vi "Get Channels from Stream Names.vi"(8 "error in (no error)":errorcluster, 10 "Stream Names":string[](array[string]), 11 "Sift Stream in":refnum<class "Sift Stream.lvclass">) -> (0 "error out":errorcluster, 2 "Channels":refnum<class "Channel.lvclass">[](array[class]), 3 "Sift Stream out":refnum<class "Sift Stream.lvclass">)   [LabVIEW 2024, in "Sift Stream.lvlib" / "Sift Stream.lvclass"]
uses:
  Sift Stream.lvclass
  <vilib>/FlexLogger/SDK/PluginSDK.lvlibp/PEFClasses/SDK/Channel/Channel.lvclass
  <vilib>/FlexLogger/SDK/PluginSDK.lvlibp/PEFClasses/SDK/Consumer Channel/Consumer Channel.lvclass
  C:/Program Files/National Instruments/LabVIEW 2024/vi.lib/FlexLogger/SDK/PluginSDK.lvlibp/PEFClasses/SDK/Channel/Channel.lvclass
  <vilib>/FlexLogger/SDK/PluginSDK.lvlibp/PEFClasses/SDK/Plugin/Get Valid Consumer Channels.vi
  <vilib>/FlexLogger/SDK/PluginSDK.lvlibp/PEFClasses/SDK/Plugin/Get Valid Producer Channels.vi
  <vilib>/FlexLogger/SDK/PluginSDK.lvlibp/PEFClasses/SDK/Plugin/Get Valid Channels.vi
  <vilib>/Utility/error.llb/Error Cluster From Error Code.vi
  <vilib>/FlexLogger/SDK/PluginSDK.lvlibp/PEFClasses/SDK/Producer Channel/Producer Channel.lvclass
  <vilib>/ErrorRing/Error Ring.xnode
  Sift Stream.lvclass/Sift Stream.ctl
  <vilib>/FlexLogger/SDK/PluginSDK.lvlibp/PEFClasses/SDK/Parameters/Parameters.lvclass
  C:/Program Files/National Instruments/LabVIEW 2024/vi.lib/FlexLogger/SDK/PluginSDK.lvlibp/PEFClasses/SDK/Consumer Channel/Consumer Channel.lvclass
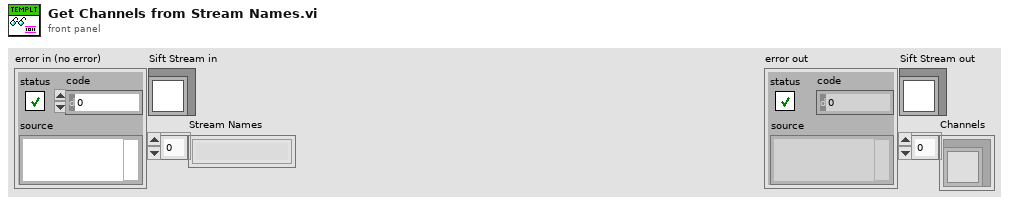
[diagram p1: front panel]
types:
  T1 = typedef "PluginSDK.lvlibp/Channel.lvclass/Data Type.ctl" = enum16{"Wfm (DBL)", "Wfm (Digital)"}
  T2 = typedef "PluginSDK.lvlibp/Parameters.lvclass/Parameter Desciption.ctl" = cluster{"Name":string, "Type":string, "Value":string}
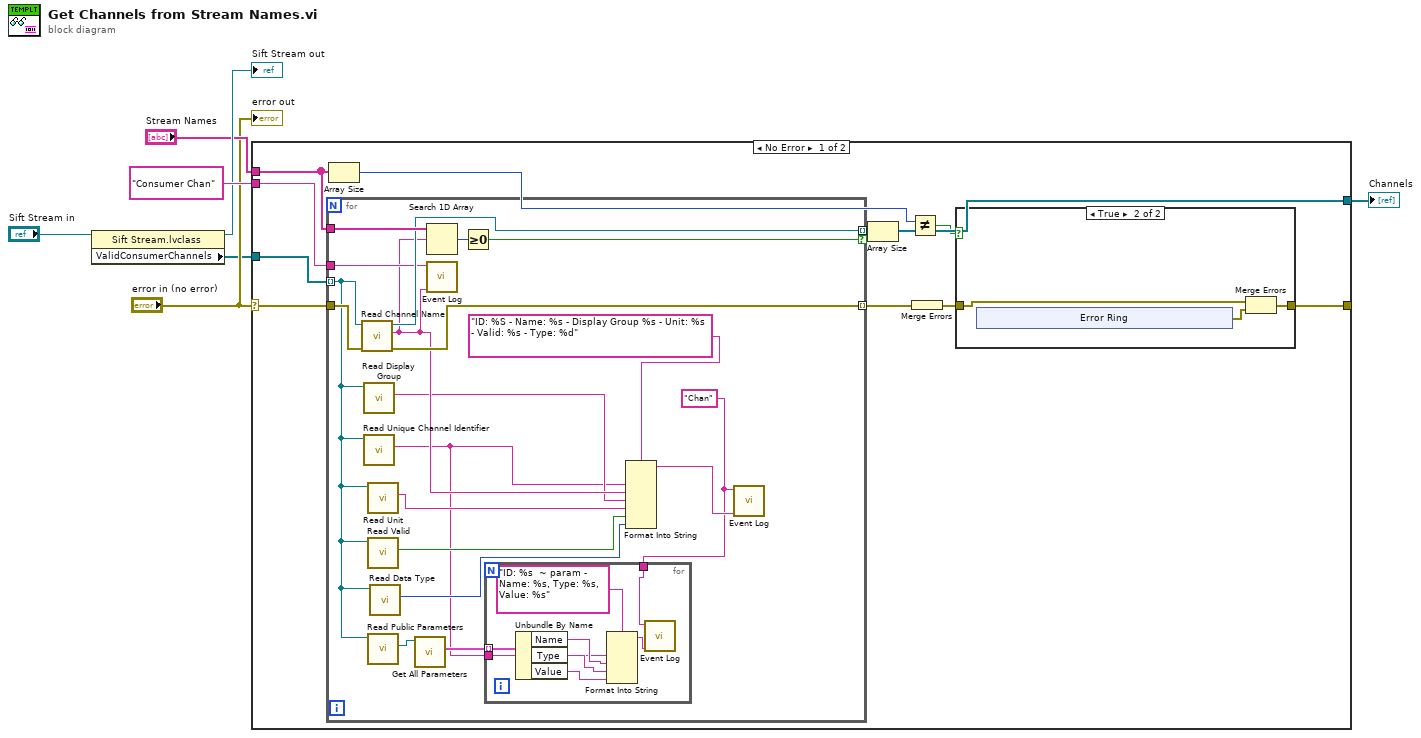
[diagram p0: block diagram]
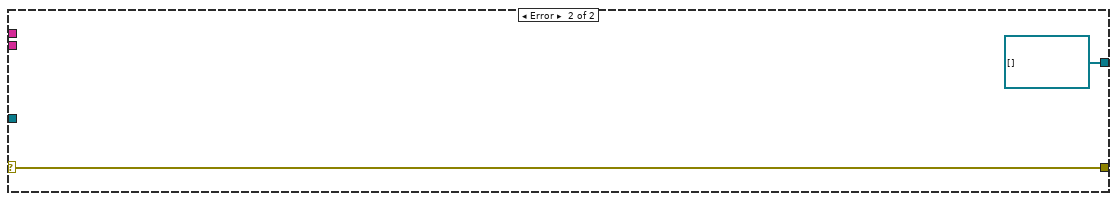
[diagram p3: hidden frame]
diagram:
  n1 = property class="Sift Stream.lvclass"(reference="Sift Stream in") -> (reference out=→"Sift Stream out":refnum<class "Sift Stream.lvclass">, "ValidConsumerChannels"=w1:refnum<class "Consumer Channel.lvclass">[])  [unwired: 1 in, 1 out]
  n2 = case shown="No Error" "error in (no error)" {
    selector: "error in (no error)" -> [w18 w56]
    tunnel: [w8 w56] -> _
    tunnel: "Stream Names" -> [w16 _]
    tunnel: [w15 refnum<class "Consumer Channel.lvclass">[] []] -> w6
    tunnel: "Consumer Chan" -> [w10 _]
    tunnel: w1 -> [w9 _]
    frame No Error {
      n3 = for {
        tunnel: w9 -> [w28] mode=indexing
        tunnel: w16 -> [w44]
        tunnel: w18 -> [w46]
        tunnel: [w45] -> w17 mode=indexing
        tunnel: [w42] -> w15 mode=indexing if=w41
        tunnel: w10 -> [w40]
        w30 = "Chan"
        n4 = call-dynamic "Read Channel Name.vi"("error in (no error)"=w46, "Channel in"=w28) -> ("error out"=w45:errorcluster, "Channel Name"=w36:string, "Channel out"=w42:refnum<class "Consumer Channel.lvclass">)  [unwired: 7 in]
        n5 = call-dynamic "Read Display Group.vi"("Channel in"=w28) -> ("Display Group"=w32:string)  [unwired: 8 in, 2 out]
        n6 = call-dynamic "Read Unique Channel Identifier.vi"("Channel in"=w28) -> ("Unique Channel Identifier"=w29:string)  [unwired: 8 in, 2 out]
        n7 = call <vilib>:"Read Unit.vi"("Channel in"=w28) -> ("Unit"=w33:string)  [unwired: 8 in, 2 out]
        n8 = call <vilib>:"Read Valid.vi"("Channel in"=w28) -> ("Valid?"=w34:bool)  [unwired: 8 in, 2 out]
        n9 = call <vilib>:"Read Public Parameters.vi"("Channel in"=w28) -> ("PluginSDK.lvlib:Parameters.lvclass"=w39:refnum<class "Parameters.lvclass">)  [unwired: 8 in, 2 out]
        n10 = call-dynamic "Read Data Type.vi"("Channel in"=w28) -> ("Data Type"=w35:T1)  [unwired: 8 in, 2 out]
        n11 = call-dynamic "Get All Parameters.vi"("Parameters in"=w39) -> ("Parameters"=w38:T2[])  [unwired: 8 in, 2 out]
        n12 = Search 1D Array(1D array=w44, element=w36) -> (index of element=w43:i32)  [unwired: 1 in]
        n13 = call "Event Log.vi"("Message"=w36, "Location"=w40) -> ()  [unwired: 10 in]
        n14 = Greater Or Equal To 0?(x=w43) -> (x >= 0?=w41:bool)
        n15 = for {
          tunnel: w38 -> [w54] mode=indexing
          tunnel: w30 -> [w50]
          tunnel: w29 -> [w47]
          n16 = Unbundle By Name(w54) -> ("Name"=w48:string, "Type"=w53:string, "Value"=w52:string)
          n17 = Format Into String(format string="ID: %s  ~ param - Name: %s, Type: %s, Value: %s", w47, w48, w53, w52) -> (resulting string=w49:string)  [unwired: 2 in, 1 out]
          n18 = call "Event Log.vi"("Message"=w49, "Location"=w50) -> ()  [unwired: 10 in]
        }
        n19 = Format Into String(format string="ID: %S - Name: %s - Display Group %s - Unit: %s - Valid: %s - Type: %d", w29, w36, w32, w33, w34, w35) -> (resulting string=w31:string)  [unwired: 2 in, 1 out]
        n20 = call "Event Log.vi"("Message"=w31, "Location"=w30) -> ()  [unwired: 10 in]
      }
      n21 = Array Size(array=w16) -> (size(s)=w14:i32)
      n22 = Array Size(array=w15) -> (size(s)=w13:i32)
      n23 = Not Equal?(x=w14, y=w13) -> (x != y?=w12:bool)
      n24 = Merge Errors(w17) -> (w11:errorcluster)
      n25 = case shown="True" w12 {
        tunnel: w11 -> [w19 w22]
        tunnel: [w19 w20] -> w8
        frame False {
        }
        frame True {
          n26 = xnode "Error Ring"() -> ("error out"=w21:errorcluster)
          n27 = Merge Errors(w22, w21) -> (w20:errorcluster)
        }
      }
    }
    frame Error {
    }
  }
  "Channels" <- w6
  "error out" <- "error in (no error)"
